vi "Get HTTP Response Code.vi"(8 "error in (no error)":errorcluster, 11 "Header":string) -> (0 "error out":errorcluster, 2 "Additional header rows":string[](array[string]), 3 "Response code":i32)   [LabVIEW 2012]
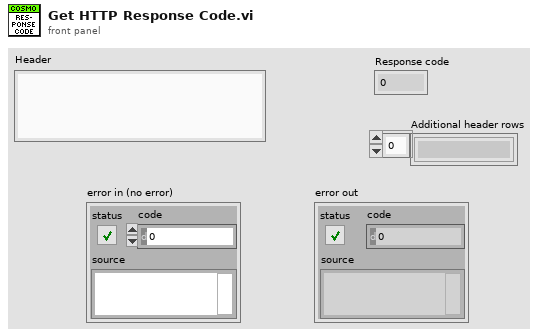
[diagram p1: front panel]
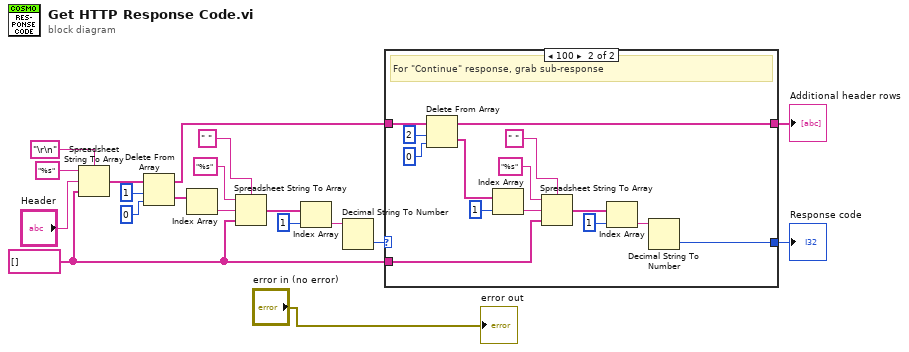
[diagram p0: block diagram]
diagram:
  w2 = string[] []
  n1 = Spreadsheet String To Array(delimiter (Tab)="\r\n", format string="%s", spreadsheet string="Header", array type (2D Dbl)=w2) -> (array=w3:string[])
  n2 = Delete From Array(array=w3, length=1, index=0) -> (deleted portion=w17:string[], array with subset deleted=w9:string[])
  n3 = Index Array(array=w17) -> (element=w16:string)  [unwired: 1 in]
  n4 = Spreadsheet String To Array(delimiter (Tab)=" ", format string="%s", spreadsheet string=w16, array type (2D Dbl)=w2) -> (array=w13:string[])
  n5 = Index Array(array=w13, index=1) -> (element=w11:string)
  n6 = Decimal String To Number(string=w11) -> (number=w10:i32)  [unwired: 2 in, 1 out]
  n7 = case shown="100" w10 {
    selector: w10 -> [w20 _]
    tunnel: w9 -> [w21 w35]
    tunnel: [w21 w32] -> w7
    tunnel: w2 -> [_ w26]
    tunnel: [w20 w22] -> w8
    frame Default {
      # "Anything but \"Continue\" (100) is pass-through"
    }
    frame 100 {
      # "For \"Continue\" response, grab sub-response"
      n8 = Delete From Array(array=w35, length=2 ("index"), index=0) -> (deleted portion=w31:string[], array with subset deleted=w32:string[])
      n9 = Index Array(array=w31, index=1) -> (element=w27:string)
      n10 = Spreadsheet String To Array(delimiter (Tab)=" ", format string="%s", spreadsheet string=w27, array type (2D Dbl)=w26) -> (array=w24:string[])
      n11 = Index Array(array=w24, index=1) -> (element=w23:string)
      n12 = Decimal String To Number(string=w23) -> (number=w22:i32)  [unwired: 2 in, 1 out]
    }
  }
  "Response code" <- w8
  "Additional header rows" <- w7
  "error out" <- "error in (no error)"
